vi "Dashboard Cell Resize.vi"(6 "Cluster":T1={"Label Font Size"=24, "Data Font Size"=36, "String Font Size"=36}, 8 "error in (no error)":errorcluster, 9 "Cluster Size:Height":u32=134, 10 "Cluster Size:Width":u32=256, 11 "ClusterRef":refnum<vi>) -> (0 "error out":errorcluster, 1 "Bounds:Area Height":u32=134, 2 "Bounds:Area Width":u32=256)   [LabVIEW 2017, in "csm-ui-support.lvlib"]
doc: "-- <b>Controls(输入控件)</b> --\n- <b>Cluster</b>:\n- <b>Cluster Size:Height</b>:\n- <b>Cluster Size:Width</b>:\n- <b>ClusterRef</b>:\n\n-- <b>Indicators(输出控件)</b> --\n- <b>Bounds:Area Height</b>:\n- <b>Bounds:Area Width</b>:\n- <b>Bounds:Area Height</b>:Indicators\n- <b>Bounds:Area Width</b>:Indicators\n- <b>Cluster Size:Height</b>:Controls\n- <b>Cluster Size:Width</b>:Controls"
uses:
  csm-ui-support.lvlib
panel:
  out "引气压力P4 2":T2={"Label"="Label", "Value"="0.00", "String"="0.00"} caption="Digital"
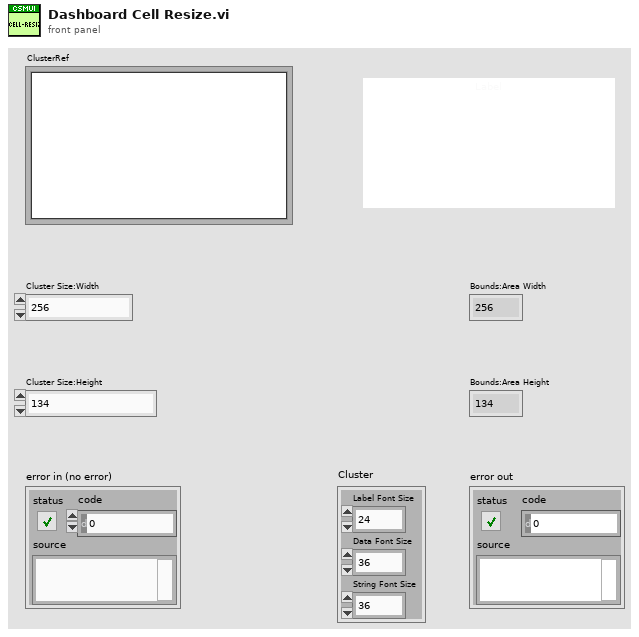
[diagram p1: front panel]
types:
  T1 = cluster{"Label Font Size":i32, "Data Font Size":i32, "String Font Size":i32}
  T2 = cluster{"Label":string, "Value":string, "String":string}
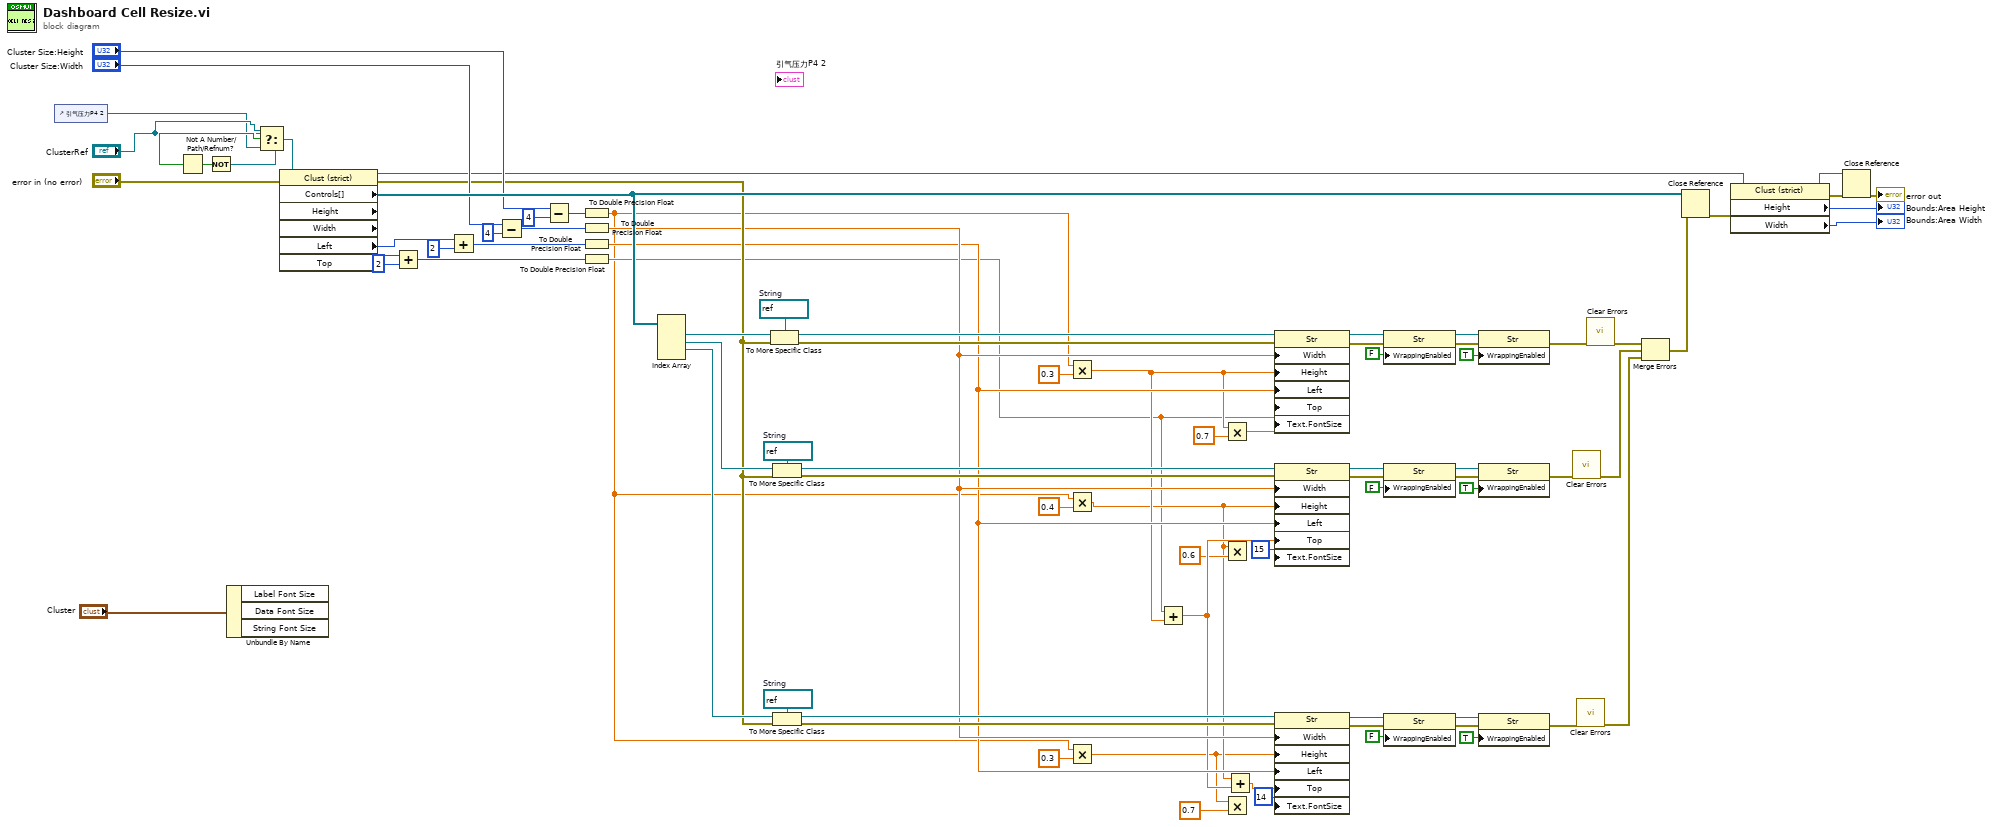
[diagram p0: block diagram]
diagram:
  w47 = refnum<vi> refnum  # String
  w78 = refnum<vi> refnum  # String
  w82 = refnum<vi> refnum  # String
  n1 = control-ref of="引气压力P4 2"() -> (w53:refnum<vi>)
  n2 = Not A Number/Path/Refnum?(number/path/refnum="ClusterRef") -> (NaN/Path/Refnum?=w3:bool)
  n3 = Not(x=w3) -> (.not. x?=w55:bool)
  n4 = Unbundle By Name("Cluster") -> ()  [unwired: 3 out]
  n5 = Select(t="ClusterRef", s=w55, f=w53) -> (s? t:f=w52:refnum<vi>)
  n6 = property on="Property Node" class="Clust (strict)" props=["Controls[]", "Height", "Width", "Left", "Top"](reference=w52, error in="error in (no error)") -> (reference out=w59:refnum<vi>, error out=w44:errorcluster, "Controls[]"=w83:refnum<vi>[], "Left"=w72:i32, "Top"=w69:i32)  [unwired: 2 out]
  n7 = Add(x=w69, y=2) -> (x+y=w50:i32)
  n8 = Add(x=w72, y=2) -> (x+y=w68:i32)
  n9 = Subtract(x="Cluster Size:Width", y=u32 4) -> (x-y=w75:u32)
  n10 = Subtract(x="Cluster Size:Height", y=u32 4) -> (x-y=w51:u32)
  n11 = To Double Precision Float(number=w51) -> (double precision float=w28:dbl)
  n12 = To Double Precision Float(number=w75) -> (double precision float=w43:dbl)
  n13 = To Double Precision Float(number=w68) -> (double precision float=w42:dbl)
  n14 = To Double Precision Float(number=w50) -> (double precision float=w31:dbl)
  n15 = Index Array(array=w83) -> (element #1=w80:refnum<vi>, element #2=w77:refnum<vi>, element #3=w45:refnum<vi>)  [unwired: 4 in, 1 out]
  n16 = To More Specific Class(target class=w82, reference=w80, error in=w44) -> (specific class reference=w81:refnum<vi>, error out=w65:errorcluster)
  n17 = To More Specific Class(target class=w78, reference=w77, error in=w44) -> (specific class reference=w79:refnum<vi>, error out=w66:errorcluster)
  n18 = To More Specific Class(target class=w47, reference=w45, error in=w44) -> (specific class reference=w46:refnum<vi>, error out=w48:errorcluster)
  n19 = Multiply(x=w28, y=0.3) -> (x*y=w37:dbl)
  n20 = Multiply(x=w28, y=0.4) -> (x*y=w33:dbl)
  n21 = Multiply(x=w28, y=0.3) -> (x*y=w30:dbl)
  n22 = Add(x=w31, y=w37) -> (x+y=w41:dbl)
  n23 = Multiply(x=w37, y=0.7) -> (x*y=w38:dbl)
  n24 = Multiply(x=w33, y=0.6) -> ()  [unwired: 1 out]
  n25 = Multiply(x=w30, y=0.7) -> ()  [unwired: 1 out]
  n26 = Add(x=w33, y=w41) -> (x+y=w49:dbl)
  n27 = property on="Property Node" class="Str"(reference=w81, error in=w65, "Width"=w43, "Height"=w37, "Left"=w42, "Top"=w31, "Text.FontSize"=w38) -> (reference out=w24:refnum<vi>, error out=w23:errorcluster)
  n28 = property on="Property Node" class="Str"(reference=w79, error in=w66, "Width"=w43, "Height"=w33, "Left"=w42, "Top"=w41, "Text.FontSize"=u32 15 ("Text.Font:Size")) -> (reference out=w12:refnum<vi>, error out=w13:errorcluster)
  n29 = property on="Property Node" class="Str"(reference=w46, error in=w48, "Width"=w43, "Height"=w30, "Left"=w42, "Top"=w49, "Text.FontSize"=u32 14 ("Text.Font:Size")) -> (reference out=w6:refnum<vi>, error out=w5:errorcluster)
  n30 = property on="Property Node" class="Str"(reference=w24, error in=w23, "WrappingEnabled"=FALSE ("Enable Wrapping")) -> (reference out=w19:refnum<vi>, error out=w20:errorcluster)
  n31 = property on="Property Node" class="Str"(reference=w12, error in=w13, "WrappingEnabled"=FALSE ("Enable Wrapping")) -> (reference out=w17:refnum<vi>, error out=w16:errorcluster)
  n32 = property on="Property Node" class="Str"(reference=w6, error in=w5, "WrappingEnabled"=FALSE ("Enable Wrapping")) -> (reference out=w7:refnum<vi>, error out=w8:errorcluster)
  n33 = property on="Property Node" class="Str"(reference=w19, error in=w20, "WrappingEnabled"=TRUE ("Enable Wrapping")) -> (error out=w18:errorcluster)  [unwired: 1 out]
  n34 = property on="Property Node" class="Str"(reference=w17, error in=w16, "WrappingEnabled"=TRUE ("Enable Wrapping")) -> (error out=w11:errorcluster)  [unwired: 1 out]
  n35 = property on="Property Node" class="Str"(reference=w7, error in=w8, "WrappingEnabled"=TRUE ("Enable Wrapping")) -> (error out=w4:errorcluster)  [unwired: 1 out]
  n36 = call <vilib>:"Clear Errors.vi"("error in (no error)"=w11) -> ("error out"=w26:errorcluster)  [unwired: 5 in, 1 out]
  n37 = call <vilib>:"Clear Errors.vi"("error in (no error)"=w4) -> ("error out"=w25:errorcluster)  [unwired: 5 in, 1 out]
  n38 = call <vilib>:"Clear Errors.vi"("error in (no error)"=w18) -> ("error out"=w27:errorcluster)  [unwired: 5 in, 1 out]
  n39 = Merge Errors(w27, w26, w25) -> (w76:errorcluster)
  n40 = Close Reference(reference=w83, error in (no error)=w76) -> (error out=w61:errorcluster)
  n41 = property on="Property Node" class="Clust (strict)"(reference=w59, error in=w61) -> (reference out=w58:refnum<vi>, error out=w60:errorcluster, "Height"=→"Bounds:Area Height":u32, "Width"=→"Bounds:Area Width":u32)
  n42 = Close Reference(reference=w58, error in (no error)=w60) -> (error out=→"error out":errorcluster)
